vi "Fetch Relative Data.vi"(0 "VISA resource name":refnum<visa-resource-name>, 1 "Zero Time Axis (T)":bool=TRUE, 5 "Latest Only (False)":bool, 11 "error in (no error)":errorcluster) -> (4 "VISA resource name out":refnum<visa-resource-name>, 6 "Relative Data":cluster{dbl[], dbl[]}(graph), 15 "error out":errorcluster)   [LabVIEW 2020, in "Keithley 648X Series.lvlib"]
doc: "Fetches the latest acquired set of relative readings.\n\n<B>Note:</B> Use this VI only with other low-level VIs. The high-level VIs automatically incorporate this functionality. This VI does not check the instrument status. If you want to check the instrument status, call the <B>Error Query</B> VI at the conclusion of the sequence."
uses:
  <instrlib>/Keithley 648X Series/Keithley 648X Series.lvlib
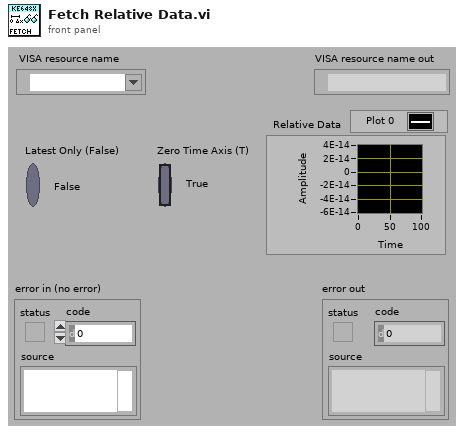
[diagram p1: front panel]
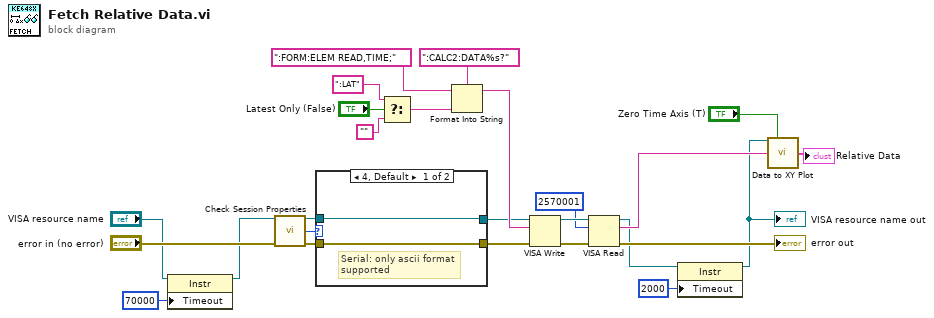
[diagram p0: block diagram]
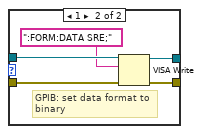
[diagram p2: hidden frame]
diagram:
  n1 = property class="Instr"(reference="VISA resource name", "Timeout"=u32 70000 ("General Settings:Timeout Value")) -> (reference out=w4:refnum<visa-resource-name>)  [unwired: 1 in, 1 out]
  n2 = call <instrlib>:"Check Session Properties.vi"("VISA resource name"=w4, "error in (no error)"="error in (no error)") -> ("VISA resource name out"=w13:refnum<visa-resource-name>, "Interface Type"=w14:u16, "error out"=w15:errorcluster)  [unwired: 10 in, 1 out]
  n3 = case shown="4, Default" w14 {
    tunnel: [w28 w33] -> w11
    tunnel: [w27 w32] -> w10
    tunnel: w15 -> [w27 w31]
    tunnel: w13 -> [w28 w30]
    frame 4, Default {
      # "Serial: only ascii format\nsupported"
    }
    frame 1 {
      # "GPIB: set data format to\nbinary"
      n4 = VISA Write(VISA resource name=w30, write buffer=":FORM:DATA SRE;", error in (no error)=w31) -> (VISA resource name out=w33:refnum<visa-resource-name>, error out=w32:errorcluster)  [unwired: 1 out]
    }
  }
  n5 = Select(t=":LAT", s="Latest Only (False)", f="") -> (s? t:f=w22:string)
  n6 = Format Into String(format string=":CALC2:DATA%s?", initial string=":FORM:ELEM READ,TIME;", w22) -> (resulting string=w21:string)  [unwired: 1 in, 1 out]
  n7 = VISA Write(VISA resource name=w11, write buffer=w21, error in (no error)=w10) -> (VISA resource name out=w19:refnum<visa-resource-name>, error out=w20:errorcluster)  [unwired: 1 out]
  n8 = VISA Read(VISA resource name=w19, byte count=u32 2570001, error in (no error)=w20) -> (VISA resource name out=w3:refnum<visa-resource-name>, read buffer=w8:string, error out=→"error out":errorcluster)  [unwired: 1 out]
  n9 = property class="Instr"(reference=w3, "Timeout"=u32 2000 ("General Settings:Timeout Value")) -> (reference out=w1:refnum<visa-resource-name>)  [unwired: 1 in, 1 out]
  "VISA resource name out" <- w1
  n10 = call <instrlib>:"Data to XY Plot.vi"("VISA resource name"=w1, "Zero Time Axis (T)"="Zero Time Axis (T)", "String of Data"=w8) -> ("XY Graph"=→"Relative Data":cluster{dbl[], dbl[]})  [unwired: 12 in]
